vi "Create API.vi"(7 "API Type (API)":refnum<class "API.lvclass">, 8 "error in (no error)":errorcluster, 11 "Task in":refnum<class "Task.lvclass">) -> (0 "error out":errorcluster, 2 "API":refnum<class "API.lvclass">, 3 "Task out":refnum<class "Task.lvclass">)   [LabVIEW 2020, in "Volatus.lvlib" / "Task.lvclass"]
uses:
  Task.lvclass
  Task.lvclass/Task.ctl
  API Provider/API Provider.lvclass
  API/API.lvclass
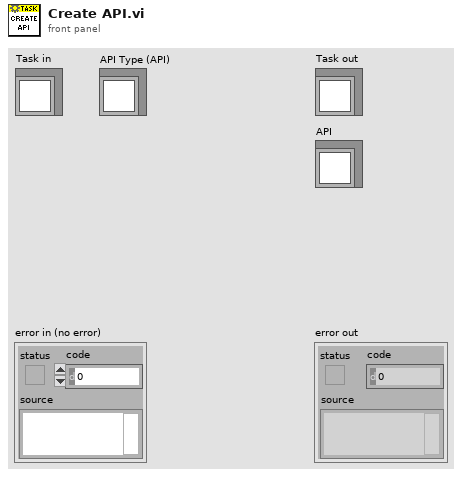
[diagram p1: front panel]
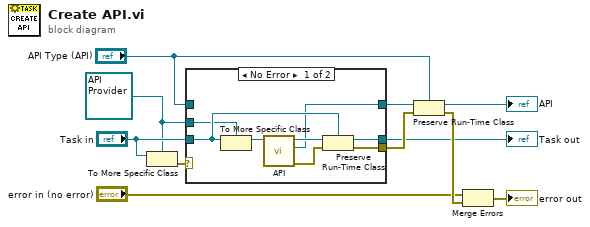
[diagram p0: block diagram]
diagram:
  w6 = refnum<class "API Provider.lvclass"> refnum ("Volatus.lvlib:API Provider.lvclass")
  n1 = To More Specific Class(target class=w6, reference="Task in") -> (error out=w9:errorcluster)  [unwired: 1 in, 1 out]
  n2 = case shown="No Error" w9 {
    tunnel: "Task in" -> [w16 w20]
    tunnel: [w15 _] -> w7
    tunnel: w6 -> [w14 _]
    tunnel: [w13 _] -> w10
    tunnel: [w12 w20] -> w5
    tunnel: "API Type (API)" -> [_ _]
    frame No Error {
      n3 = To More Specific Class(target class=w14, reference=w16) -> (specific class reference=w19:refnum<class "API Provider.lvclass">)  [unwired: 1 in, 1 out]
      n4 = call-dynamic "API.vi"("API Provider in"=w19) -> ("error out"=w17:errorcluster, "API"=w15:refnum<class "API.lvclass">, "API Provider out"=w18:refnum<class "API Provider.lvclass">)  [unwired: 8 in]
      n5 = Preserve Run-Time Class(object in=w18, error in=w17, 2:w16) -> (object out=w12:refnum<class "Task.lvclass">, error out=w13:errorcluster)
    }
    frame Error {
      # "Not API Provider, ignore."
    }
  }
  "Task out" <- w5
  n6 = Preserve Run-Time Class(object in=w7, error in=w10, 2:"API Type (API)") -> (object out=→"API":refnum<class "API.lvclass">, error out=w11:errorcluster)
  n7 = Merge Errors("error in (no error)", w11) -> (→"error out":errorcluster)
